vi "Practica1.vi"() -> ()   [LabVIEW 2021]
uses:
  <vilib>/imath/engines/lvmath2/RunTimeEngine/Managers/WorkSpace/UID Generator.vi
  <vilib>/imath/engines/lvmath2/RunTimeEngine/ArithmeticOperatorToken/NIMS_ArithmeticOperator_power(S).vi
  <instcachedir>/0/NIMS_ArithmeticOperator_power(S)_149E20C93FA648E196B974450BC90546.lvgen/NIMS_ArithmeticOperator_power(S)_149E20C93FA648E196B974450BC90546_010.vi
  <vilib>/imath/engines/lvmath2/RunTimeEngine/RunTimeType/NIMS_RunTimeType_From StrictType (excl LVString).vi
  <instcachedir>/0/NIMS_RunTimeType_From StrictType (excl LVString)_F2DF8362C4A748C4A5A87B97B2A722F9.lvgen/NIMS_RunTimeType_From StrictType (excl LVString)_F2DF8362C4A748C4A5A87B97B2A722F9_000.vi
  <vilib>/imathl/engines/lvmath/Functions/Error Handling/Create Error.vi
  <vilib>/imath/engines/lvmath2/RunTimeEngine/LocalVariableDefStatement/MC_LocalVariableDefStatement_Display.vi
  <vilib>/imath/engines/lvmath2/RunTimeEngine/BuiltInFunctions/sin/NIMS_sin(C).vi
  <instcachedir>/0/NIMS_sin(C)_EF49EB6613814DD5AA1481177C690C0D.lvgen/NIMS_sin(C)_EF49EB6613814DD5AA1481177C690C0D_001.vi
  <vilib>/imath/engines/lvmath2/RunTimeEngine/BuiltInFunctions/cos/NIMS_cos(C).vi
  <instcachedir>/0/NIMS_cos(C)_035A4A914C7C4DF2869F8321D2939141.lvgen/NIMS_cos(C)_035A4A914C7C4DF2869F8321D2939141_001.vi
  <vilib>/imath/engines/lvmath2/RunTimeEngine/BuiltInFunctions/conv/NIMS_conv(V,V).vi
  <instcachedir>/0/NIMS_conv(V,V)_D3E194F2B5174935BB2368CEB7AAC5A9.lvgen/NIMS_conv(V,V)_D3E194F2B5174935BB2368CEB7AAC5A9_000.vi
  <vilib>/imath/engines/lvmath2/RunTimeEngine/ErrorHandling/NIMS_Error From Error Code.vi
  <vilib>/imath/engines/lvmath2/RunTimeEngine/IndexRead/NIMS V(S).vi
  <instcachedir>/0/NIMS V(S)_0488751826AF41519A22953C041130DC.lvgen/NIMS V(S)_0488751826AF41519A22953C041130DC_003.vi
  <vilib>/imath/engines/lvmath2/RunTimeEngine/ErrorHandling/NIMS_Create Error From Enums.vi
  <vilib>/imath/engines/lvmath2/RunTimeEngine/BuiltInFunctions/inv/NIMS_inv(GM).vi
  <instcachedir>/0/NIMS_inv(GM)_A6DF8FE880224208AACFE4CF9F659502.lvgen/NIMS_inv(GM)_A6DF8FE880224208AACFE4CF9F659502_001.vi
  <vilib>/imath/engines/lvmath2/RunTimeEngine/ArithmeticOperatorToken/NIMS_ArithmeticOperator_multmx(M,CV).vi
  <instcachedir>/0/NIMS_ArithmeticOperator_multmx(M,CV)_EA5705981BE742938BF830F3274AE397.lvgen/NIMS_ArithmeticOperator_multmx(M,CV)_EA5705981BE742938BF830F3274AE397_002.vi
  <vilib>/imath/engines/lvmath2/RunTimeEngine/IndexRead/NIMS M(S).vi
  <instcachedir>/0/NIMS M(S)_B826C018497E4940AE96BD27B540B6FB.lvgen/NIMS M(S)_B826C018497E4940AE96BD27B540B6FB_004.vi
  <vilib>/imath/engines/lvmath2/RunTimeEngine/Managers/SymbolTable/Clear UID.vi
  <vilib>/imath/engines/lvmath2/RunTimeEngine/NodeEndStatement/NIMS_NodeEndStatement_Output.vi
  <instcachedir>/0/NIMS_NodeEndStatement_Output_53EC0D466D134D7ABD903AC30B43404B.lvgen/NIMS_NodeEndStatement_Output_53EC0D466D134D7ABD903AC30B43404B_001.vi
  <instcachedir>/0/NIMS_NodeEndStatement_Output_53EC0D466D134D7ABD903AC30B43404B.lvgen/NIMS_NodeEndStatement_Output_53EC0D466D134D7ABD903AC30B43404B_010.vi
  <instcachedir>/0/NIMS_NodeEndStatement_Output_53EC0D466D134D7ABD903AC30B43404B.lvgen/NIMS_NodeEndStatement_Output_53EC0D466D134D7ABD903AC30B43404B_009.vi
  <vilib>/imath/engines/lvmath2/RunTimeEngine/ErrorHandling/NIMS_Finalize Error.vi
  <vilib>/imath/engines/lvmath2/RunTimeEngine/Managers/SymbolTable/NIMS_WorkSpace.lvlib
panel:
  in  "Nivel de perturbación":dbl(slide) scale=0.0..10.0
  in  "Perturbación":bool
  out "Error":dbl
  in  "Selector":bool caption="Boolean"
  in  "a1":dbl=-0.678
  in  "b2":dbl=0.0168
  in  "b1":dbl=0.4592
  in  "Tm":dbl=0.07
  in  "Mp":dbl=10.0
  in  "tss":dbl=0.6
  in  "stop":bool
  in  "Set Point":dbl
  out "Sistema Controlado":T1(graph)
  # "Laboratorio Control Avanzado"
  # "Diseno de Controladores PI y PID por Asignación de Polos"
  # "Andrés Felipe Garavito González"
  # "Esteban Vásquez Cano"
  # "PID"
  # "PI"
  # "z    +"
  # "HGp(z) = ----------------------------------"
  # "z^2   +"
  # "z"
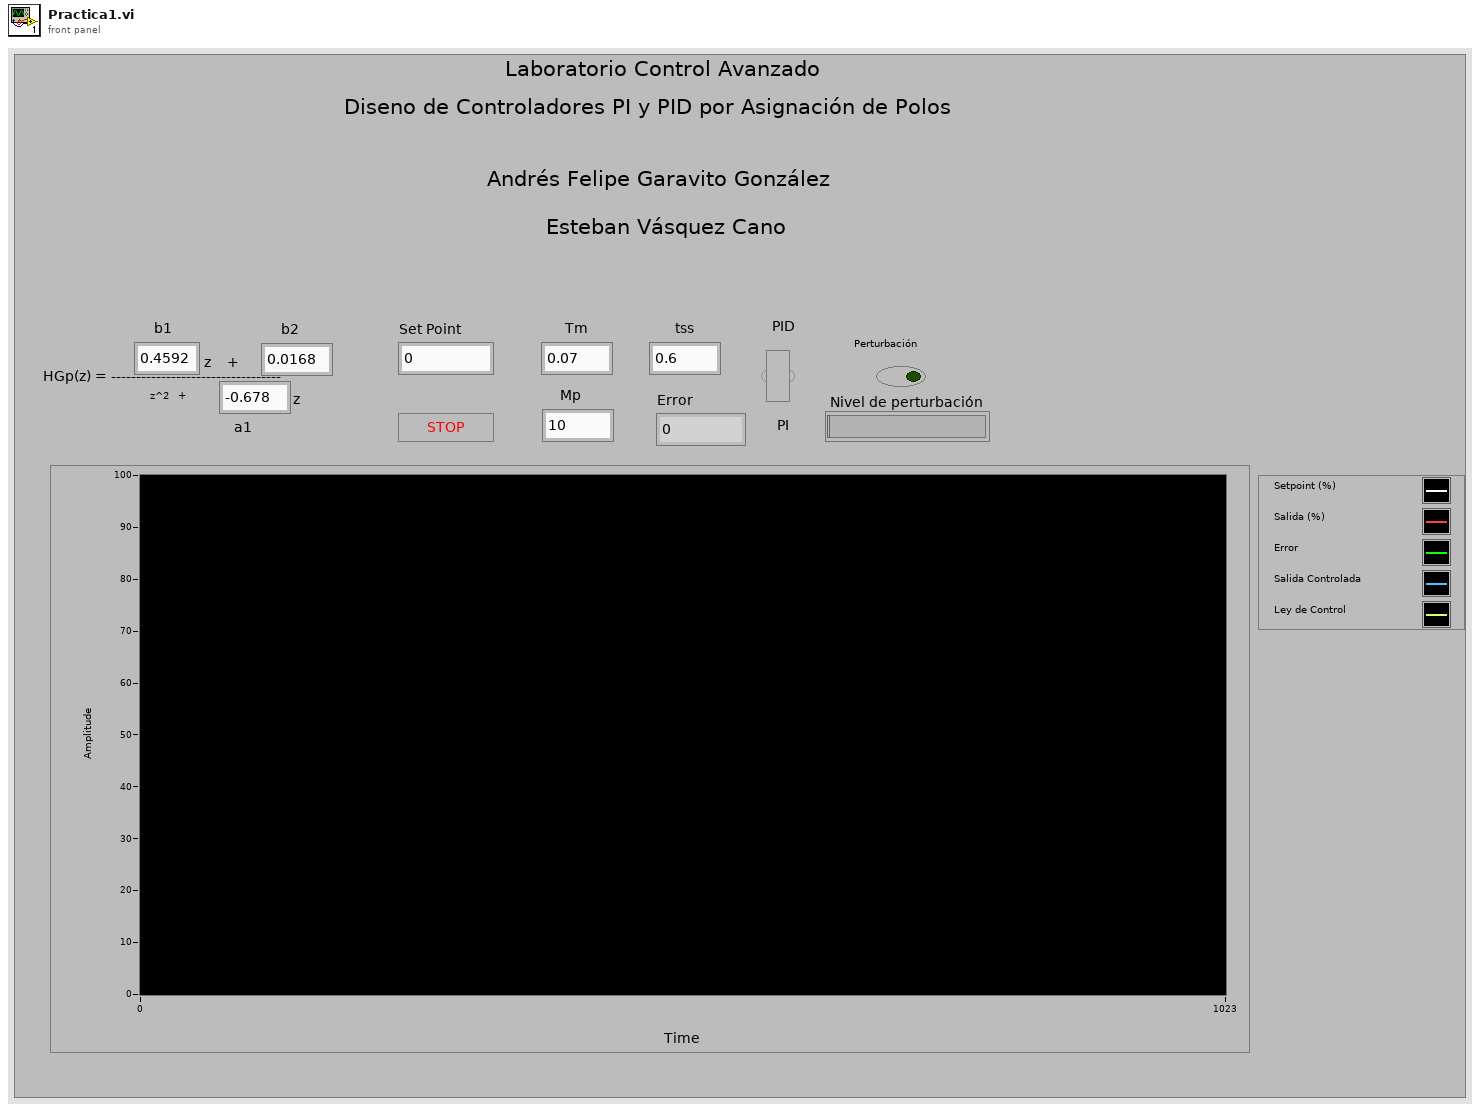
[diagram p1: front panel]
types:
  T1 = cluster{"Set Point U(k)":dbl, "yk":dbl, "Error":dbl, "ykc":dbl, "mk":dbl}
  T2 = cluster{"Set Point":dbl, "yk":dbl, cdb, "ykc":cdb, "mk":cdb}
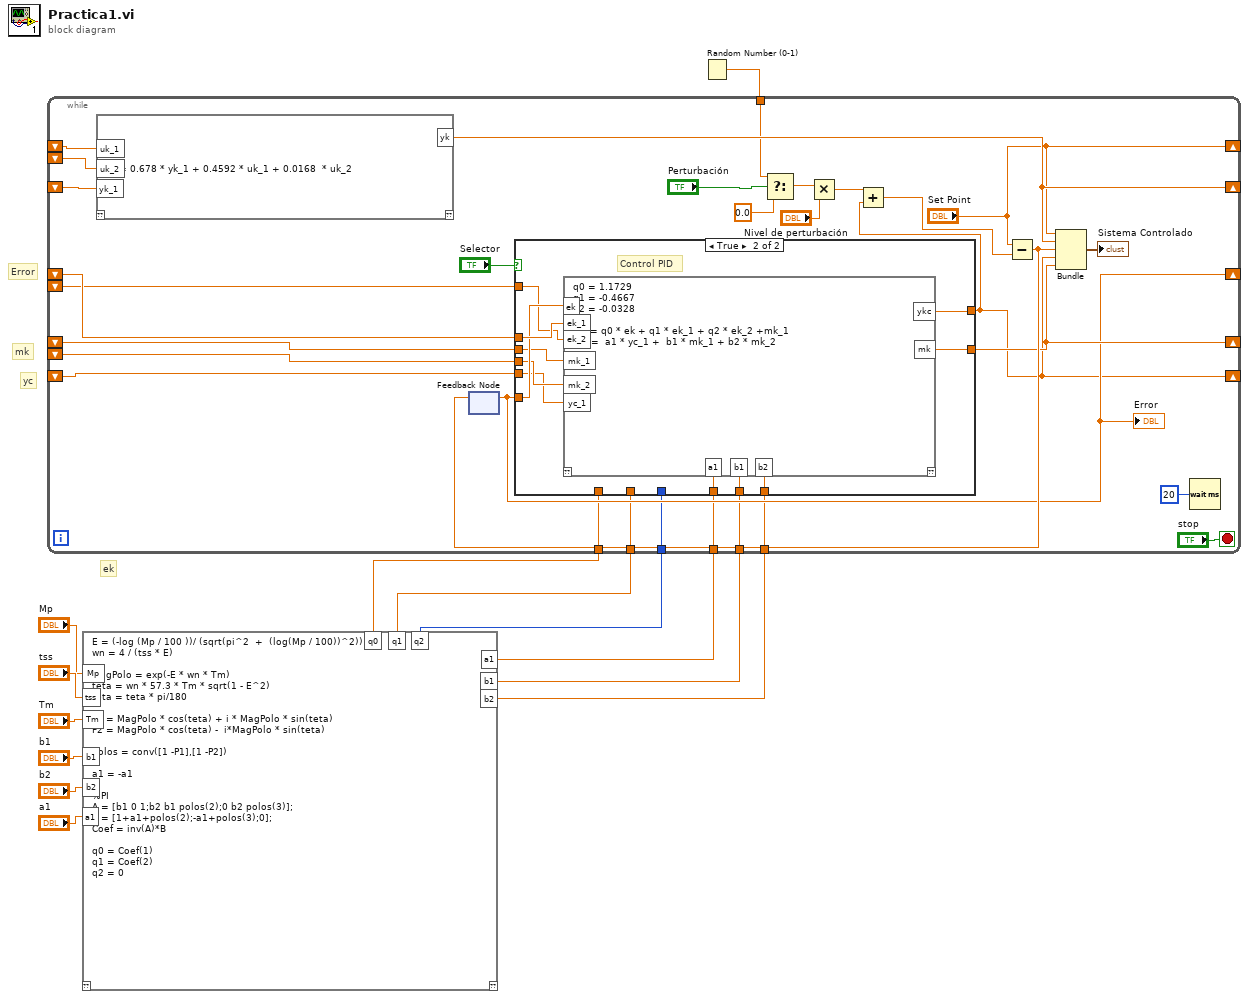
[diagram p0: block diagram]
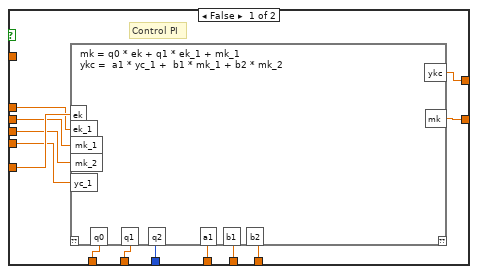
[diagram p2: hidden frame]
diagram:
  # "Error"
  # "yc"
  # "mk"
  # "ek"
  n1 = mathscript code="E = (-log (Mp / 100 ))/ (sqrt(pi^2  +  (log(Mp / 100))^2))\nwn = 4 / (tss * E)\n\nMagPolo = exp(-E * wn * Tm)\nteta = wn * 57.3 * Tm * sqrt(1 - E^2)\nteta = teta * pi/180\n\nP1 = MagPolo * cos(teta) + i * MagPolo * sin(teta)\nP2 = MagPolo * cos(teta) -  i*MagPolo * sin(teta)\n\npolos = conv([1 -P1],[1 -P2])\n\na1 = -a1\n\n%PI\nA = [b1 0 1;b2 b1 polos(2);0 b2 polos(3)];\nB = [1+a1+polos(2);-a1+polos(3);0];\nCoef = inv(A)*B\n\nq0 = Coef(1)\nq1 = Coef(2)\nq2 = 0"("Mp"="Mp", "tss"="tss", "Tm"="Tm", "b1"="b1", "b2"="b2", "a1"="a1") -> ("q0"=w7:cdb, "q1"=w6:cdb, "q2"=w5:i32, "a1"=w4:dbl, "b1"=w3:dbl, "b2"=w2:dbl)  [unwired: 1 in, 1 out]
  n2 = Random Number (0-1)() -> (number: 0 to 1=w1:dbl)
  n3 = while {
    shift-right: [w41] -> _
    shift-left: _ -> [w42]
    shift-right: ["Set Point"] -> _
    shift-left: _ -> [w44]
    shift-left: _ -> [w43]
    shift-right: [w30] -> _
    shift-left: _ -> [w34]
    shift-left: _ -> [w33]
    shift-right: [w17] -> _
    shift-left: _ -> [w32]
    shift-right: [w29] -> _
    shift-left: _ -> [w35]
    tunnel: w7 -> [w28]
    tunnel: w6 -> [w27]
    tunnel: w5 -> [w26]
    tunnel: w4 -> [w25]
    tunnel: w3 -> [w24]
    tunnel: w2 -> [w23]
    shift-left: _ -> [w22]
    tunnel: w1 -> [w15]
    stop <- "stop" stop-if-true
    n4 = mathscript code="yk = 0.678 * yk_1 + 0.4592 * uk_1 + 0.0168  * uk_2"("yk_1"=w42, "uk_1"=w44, "uk_2"=w43) -> ("yk"=w41:dbl)  [unwired: 1 in, 1 out]
    n5 = feedback #1() -> (w29:cdb)  [unwired: 1 in]
    "Error" <- w29
    n6 = case shown="True" "Selector" {
      tunnel: w29 -> [w57 w146]
      tunnel: w35 -> [w56 w147]
      tunnel: w34 -> [w55 w144]
      tunnel: w33 -> [w54 w143]
      tunnel: w32 -> [w53 w142]
      tunnel: [w51 w152] -> w17
      tunnel: [w52 w151] -> w30
      tunnel: w28 -> [w50 _]
      tunnel: w27 -> [w49 _]
      tunnel: w26 -> [w48 _]
      tunnel: w25 -> [w47 w150]
      tunnel: w24 -> [w46 w149]
      tunnel: w23 -> [w45 w148]
      tunnel: w22 -> [_ w145]
      frame False {
        # "Control PI"
        n7 = mathscript code="mk = q0 * ek + q1 * ek_1 + mk_1\nykc =  a1 * yc_1 +  b1 * mk_1 + b2 * mk_2"("q1"=w49, "q0"=w50, "ek"=w57, "ek_1"=w56, "mk_1"=w55, "mk_2"=w54, "yc_1"=w53, "q2"=w48, "a1"=w47, "b1"=w46, "b2"=w45) -> ("mk"=w52:cdb, "ykc"=w51:cdb)  [unwired: 1 in, 1 out]
      }
      frame True {
        # "Control PID"
        n8 = mathscript code="q0 = 1.1729\nq1 = -0.4667\nq2 = -0.0328\n\nmk = q0 * ek + q1 * ek_1 + q2 * ek_2 +mk_1\nykc =  a1 * yc_1 +  b1 * mk_1 + b2 * mk_2"("a1"=w150, "b1"=w149, "b2"=w148, "ek"=w146, "ek_1"=w147, "ek_2"=w145, "mk_1"=w144, "mk_2"=w143, "yc_1"=w142) -> ("mk"=w151:cdb, "ykc"=w152:cdb)  [unwired: 1 in, 1 out]
      }
    }
    n9 = Select(t=w15, s="Perturbación", f=0.0) -> (s? t:f=w19:dbl)
    n10 = Multiply(x=w19, y="Nivel de perturbación") -> (x*y=w18:dbl)
    n11 = Add(x=w18, y=w17) -> (x+y=w16:cdb)
    n12 = Subtract(x="Set Point", y=w16) -> (x-y=w37:cdb)
    n13 = feedback-in #1(w37) -> ()
    n14 = Bundle("Set Point"="Set Point", "yk"=w41, w37, "ykc"=w17, "mk"=w30) -> (→"Sistema Controlado":T2)  [unwired: 1 in]
    n15 = Wait (ms)(milliseconds to wait=u32 20) -> ()  [unwired: 1 out]
  }
